vi "DBL to String.vi"(10 "Format String":string, 11 "Promise":refnum<class "Promise.lvclass">) -> ()   [LabVIEW 2020, in "Futures-Examples.lvlib"]
uses:
  Futures-Examples.lvlib
  Promises/Promise/Promise.lvclass
  DoubleValue/DoubleValue.lvclass
  StringValue/StringValue.lvclass
  876598b3-b805-474f-ae4f-c8c280077482.vi
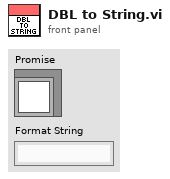
[diagram p1: front panel]
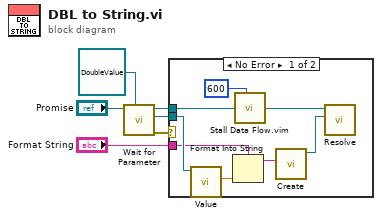
[diagram p0: block diagram]
diagram:
  n1 = call "Wait for Parameter.vi"("Param Type (Default)"=refnum<class "DoubleValue.lvclass"> refnum ("Futures-Examples.lvlib:DoubleValue.lvclass"), "Promise in"="Promise") -> ("error out"=w4:errorcluster, "Parameter"=w3:refnum<class "DoubleValue.lvclass">, "Promise out"=w2:refnum<class "Promise.lvclass">)  [unwired: 7 in]
  n2 = case shown="No Error" w4 {
    tunnel: w3 -> [w14 _]
    tunnel: w2 -> [w10 _]
    tunnel: "Format String" -> [w13 _]
    frame No Error {
      n3 = call "Value.vi"("DoubleValue in"=w14) -> ("Value"=w12:dbl)  [unwired: 10 in]
      n4 = Format Into String(format string=w13, w12) -> (resulting string=w11:string)  [unwired: 2 in, 1 out]
      n5 = call "Stall Data Flow.vim"("value in"=w10, "milliseconds to wait"=u32 600) -> ("value out"=w8:refnum<class "Promise.lvclass">)  [unwired: 1 out]
      n6 = call "Create.vi"("Value"=w11) -> ("StringValue out"=w9:refnum<class "StringValue.lvclass">)  [unwired: 10 in]
      n7 = call "Resolve.vi"("Result"=w9, "Promise in"=w8) -> ()  [unwired: 8 in, 2 out]
    }
    frame Error {
    }
  }
